vi "TodayDate.vi"(8 "error in (no error)":errorcluster, 11 "Calendar in":refnum<class "Calendar.lvclass">) -> (0 "error out":errorcluster, 3 "Calendar (dup)":refnum<class "Calendar.lvclass">)   [LabVIEW 2020, in "Calendar.lvclass"]
uses:
  Calendar.lvclass
  Calendar.lvclass/Calendar.ctl
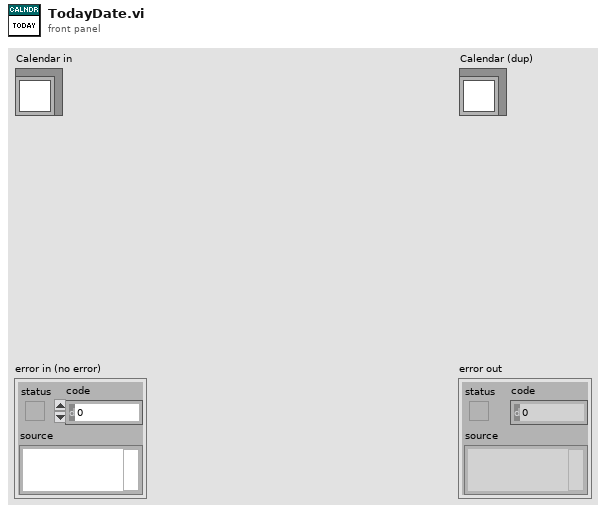
[diagram p1: front panel]
types:
  T1 = typedef "Calendar.lvclass/State Data.ctl" = cluster{"Current Date":timestamp, "First Day of Week":T2, "Color":cluster{"Selector Background":u32, "Selector Text":u32, "Days of Week Background":u32, "Days of Week Text":u32, "Calendar Background":u32, "Calendar Text":u32, "Calendar Selection Background":u32, "Calendar Selection Text":u32}, "Visible":cluster{"Today Selector Visible":bool, "Month-Year Selector Visible":bool}}
  T2 = typedef "Calendar.lvclass/DaysOfWeek.ctl" = enum16{"Sunday", "Monday", "Tuesday", "Wednesday", "Thursday", "Friday", "Saturday"}
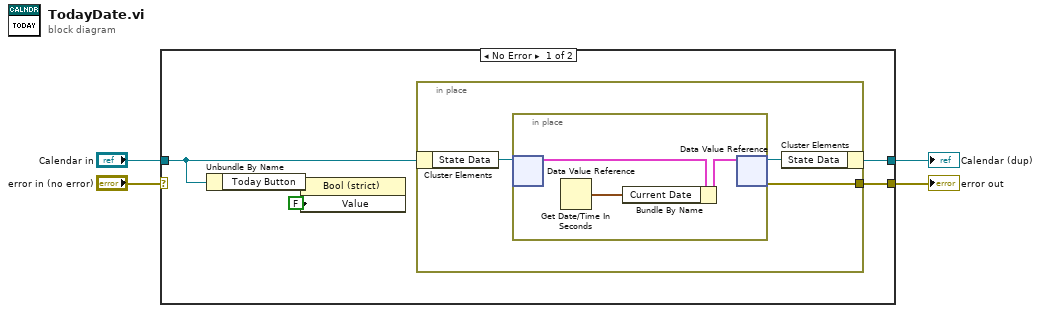
[diagram p0: block diagram]
diagram:
  n1 = case shown="No Error" "error in (no error)" {
    selector: "error in (no error)" -> [_ w17]
    tunnel: [w8 w17] -> w3
    tunnel: [w9 w16] -> w1
    tunnel: "Calendar in" -> [w5 w16]
    frame No Error {
      n2 = Unbundle By Name(w5) -> ("Today Button"=w7:refnum<vi>)
      n3 = property class="Bool (strict)"(reference=w7, "Value"=FALSE) -> ()  [unwired: 1 in, 2 out]
      n4 = in-place {
        in-place-border: [w10] -> w8
        n5 = in-place-cluster #1(w5) -> ("State Data"=w12:refnum<data-value>)
        n6 = in-place {
          n7 = in-place-dvr #2(w12) -> (w15:T1)  [unwired: 1 out]
          n8 = Get Date/Time In Seconds() -> (seconds since 1Jan1904=w13:timestamp)
          n9 = Bundle By Name(cluster=w15, "Current Date"=w13) -> (w14:T1)
          n10 = in-place-dvr #2(w14) -> (w11:refnum<data-value>, w10:errorcluster)
        }
        n11 = in-place-cluster #1("State Data"=w11) -> (w9:refnum<class "Calendar.lvclass">)
      }
    }
    frame Error {
    }
  }
  "error out" <- w3
  "Calendar (dup)" <- w1
